vi "Format Vacuum Test Result Table.vi"(10 "Test Configuration":T1, 11 "Test Results":T8) -> (2 "Failure Indexes":i32[](array[numeric]), 3 "Vacuum Results":string[][](array[string]))   [LabVIEW 2014]
uses:
  Tests/Controls/Test Results.ctl
  Tests/Controls/Step Result.ctl
  Tests/Controls/Test Configuration.ctl
  Tests/Controls/Vacuum Test.ctl
  Tests/Controls/Test Timing.ctl
  Tests/Controls/Vaccum Thresholds.ctl
  Tests/Controls/Helium Test.ctl
  Tests/Controls/Helium Thresholds.ctl
  Tests/Controls/Functional Test.ctl
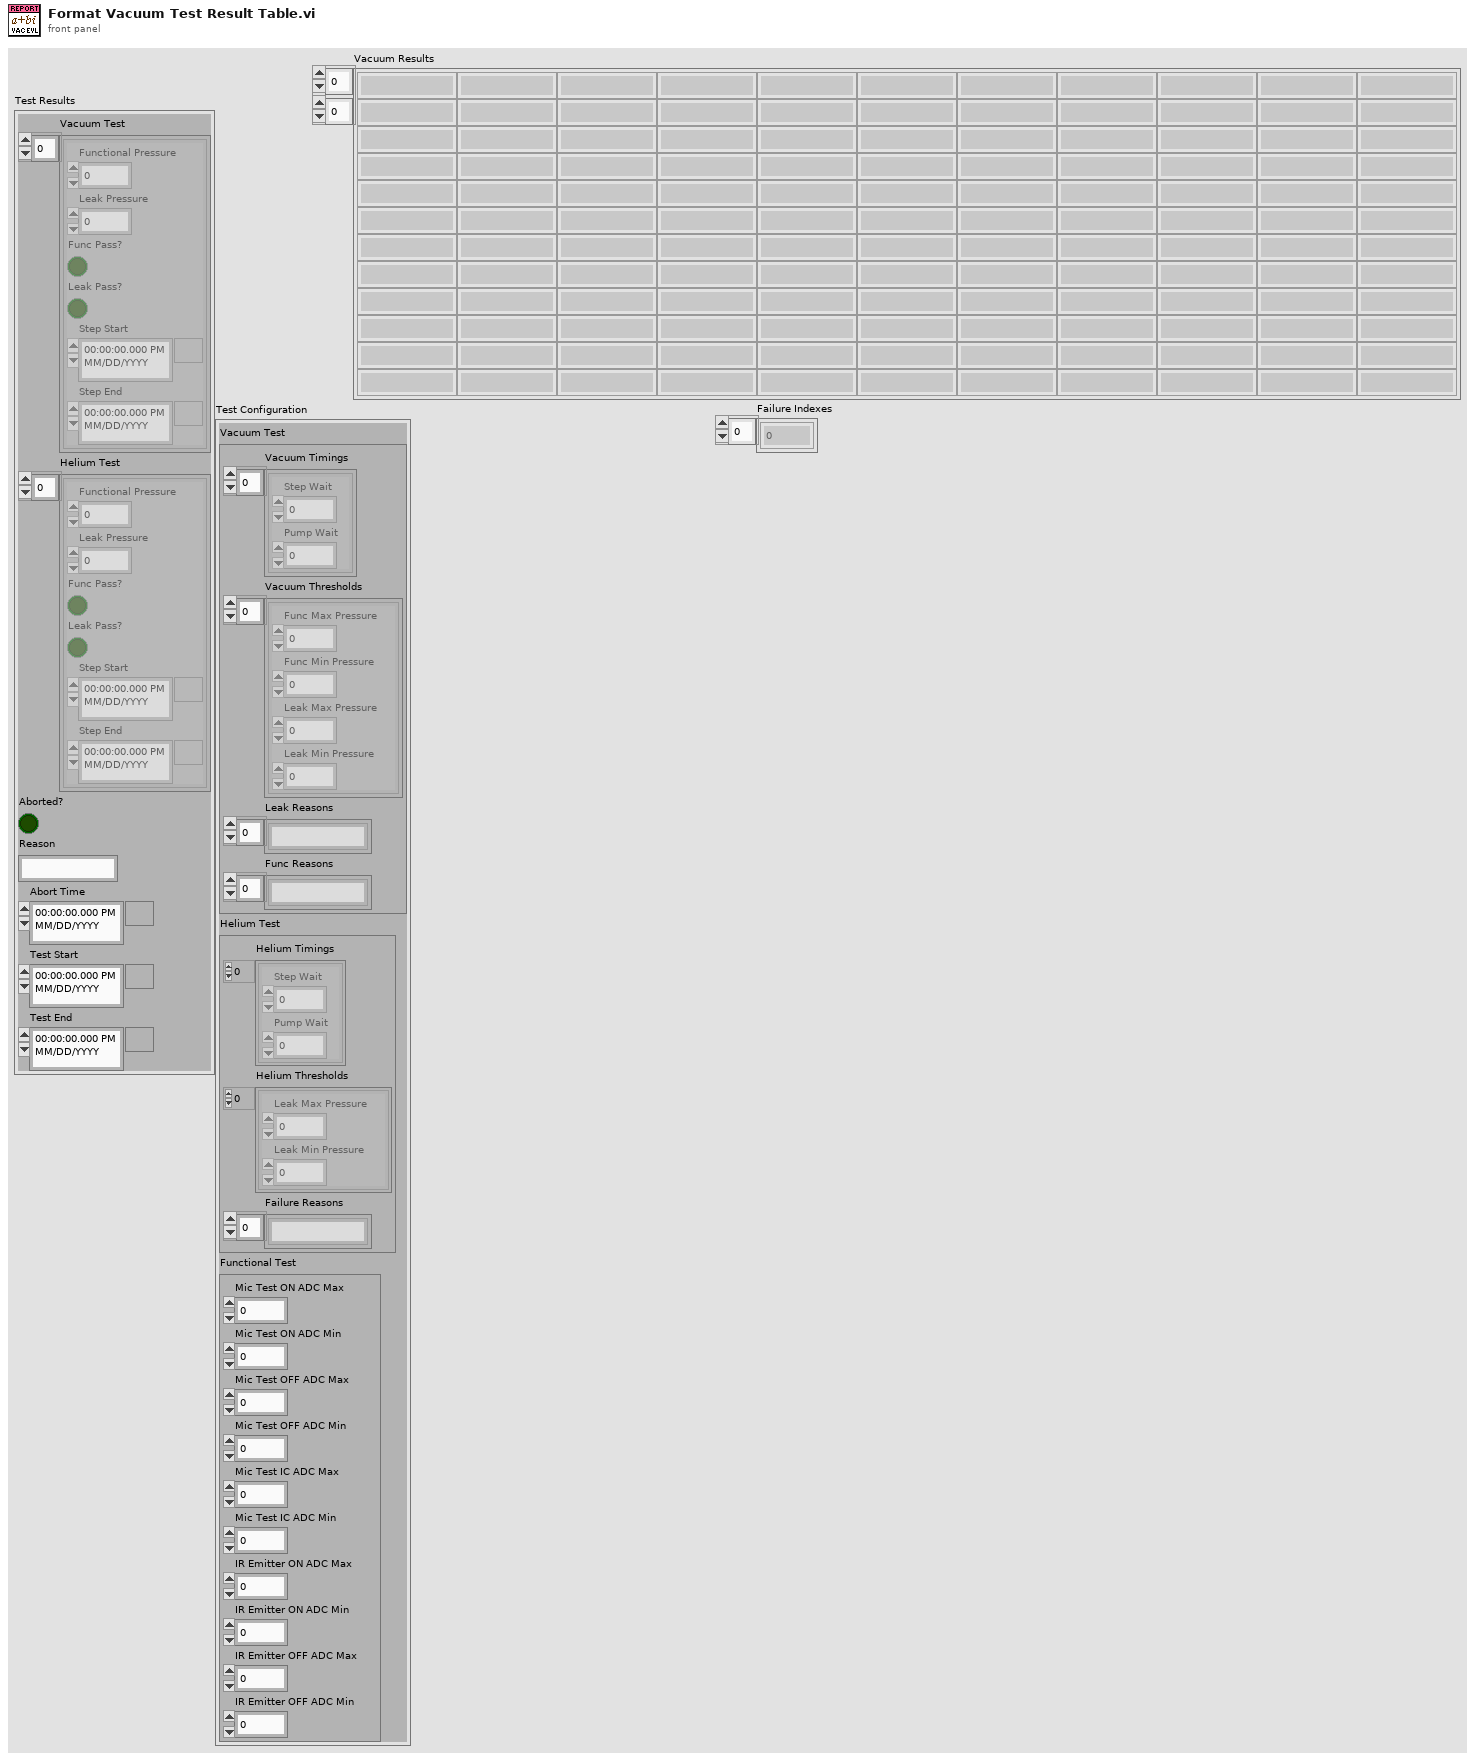
[diagram p1: front panel]
types:
  T1 = typedef "Test Configuration.ctl" = cluster{"Vacuum Test":T2, "Helium Test":T5, "Functional Test":T7}
  T2 = typedef "Vacuum Test.ctl" = cluster{"Vacuum Timings":T3[], "Vacuum Thresholds":T4[], "Leak Reasons":string[], "Func Reasons":string[]}
  T3 = typedef "Test Timing.ctl" = cluster{"Step Wait":dbl, "Pump Wait":dbl}
  T4 = typedef "Vaccum Thresholds.ctl" = cluster{"Func Max Pressure":dbl, "Func Min Pressure":dbl, "Leak Max Pressure":dbl, "Leak Min Pressure":dbl}
  T5 = typedef "Helium Test.ctl" = cluster{"Helium Timings":T3[], "Helium Thresholds":T6[], "Failure Reasons":string[]}
  T6 = typedef "Helium Thresholds.ctl" = cluster{"Leak Max Pressure":dbl, "Leak Min Pressure":dbl}
  T7 = typedef "Functional Test.ctl" = cluster{"Mic Test ON ADC Max":dbl, "Mic Test ON ADC Min":dbl, "Mic Test OFF ADC Max":dbl, "Mic Test OFF ADC Min":dbl, "Mic Test IC ADC Max":dbl, "Mic Test IC ADC Min":dbl, "IR Emitter ON ADC Max":dbl, "IR Emitter ON ADC Min":dbl, "IR Emitter OFF ADC Max":dbl, "IR Emitter OFF ADC Min":dbl}
  T8 = typedef "Test Results.ctl" = cluster{"Vacuum Test":T9[], "Helium Test":T9[], "Aborted?":bool, "Reason":string, "Abort Time":timestamp, "Test Start":timestamp, "Test End":timestamp}
  T9 = typedef "Step Result.ctl" = cluster{"Functional Pressure":dbl, "Leak Pressure":dbl, "Func Pass?":bool, "Leak Pass?":bool, "Step Start":timestamp, "Step End":timestamp}
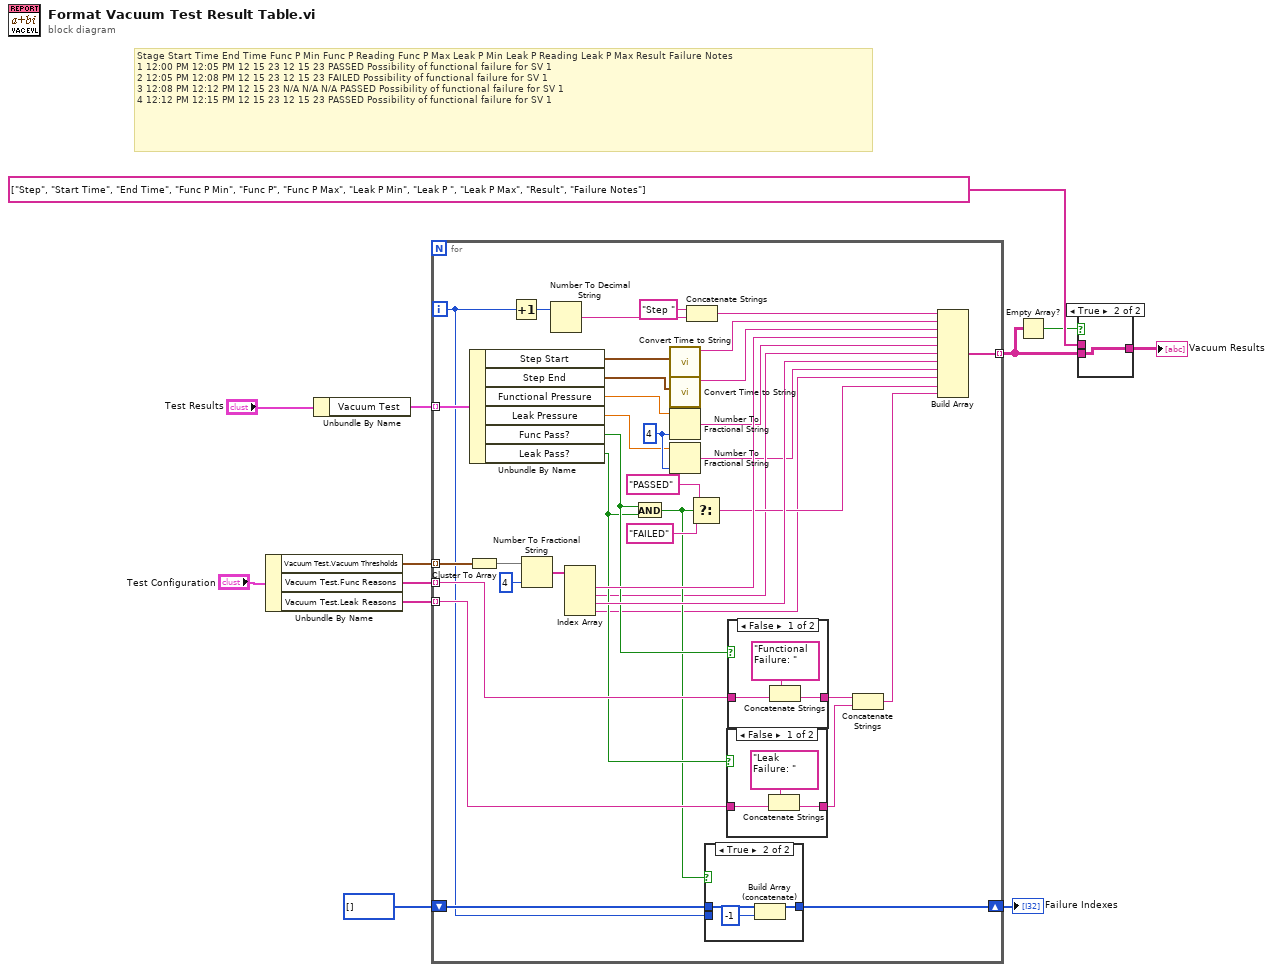
[diagram p0: block diagram]
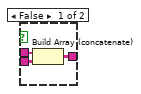
[diagram p2: hidden frame]
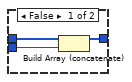
[diagram p3: hidden frame]
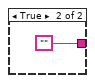
[diagram p4: hidden frame]
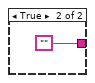
[diagram p5: hidden frame]
diagram:
  # "Stage\tStart Time\tEnd Time\tFunc P Min\tFunc P Reading\tFunc P Max\tLeak P Min\tLeak P Reading\tLeak P Max\tResult\tFailure Notes\n1\t12:00 PM\t12:05 PM\t12\t15\t23\t12\t15\t23\tPASSED\tPossibility of functional failure for SV 1\n2\t12:05 PM\t12:08 PM\t12\t15\t23\t12\t15\t23\tFAILED\tPossibility of functional failure for SV 1\n3\t12:08 PM\t12:12 PM\t12\t15\t23\tN/A\tN/A\tN/A\tPASSED\tPossibility of functional failure for SV 1\n4\t12:12 PM\t12:15 PM\t12\t15\t23\t12\t15\t23\tPASSED\tPossibility of functional failure for SV 1"
  n1 = Unbundle By Name("Test Configuration") -> ("Vacuum Test.Vacuum Thresholds"=w10:T4[], "Vacuum Test.Func Reasons"=w9:string[], "Vacuum Test.Leak Reasons"=w8:string[])
  n2 = Unbundle By Name("Test Results") -> ("Vacuum Test"=w11:T9[])
  n3 = for {
    tunnel: w11 -> [w49] mode=indexing
    tunnel: w10 -> [w45] mode=indexing
    tunnel: w9 -> [w27] mode=indexing
    tunnel: w8 -> [w22] mode=indexing
    tunnel: [w24] -> w3 mode=indexing
    shift-right: [w17] -> w4
    shift-left: i32[] [] -> [w19]
    i -> [w18]
    w33 = i16 4 ("precision (6)")
    n4 = Cluster To Array(cluster=w45) -> (array=w44:dbl[])
    n5 = Unbundle By Name(w49) -> ("Step Start"=w47:timestamp, "Step End"=w46:timestamp, "Functional Pressure"=w41:dbl, "Leak Pressure"=w32:dbl, "Func Pass?"=w28:bool, "Leak Pass?"=w23:bool)
    n6 = Increment(x=w18) -> (x+1=w48:i32)
    n7 = Number To Fractional String(number=w44, precision (6)=i16 4) -> (F-format string=w42:string[])  [unwired: 2 in]
    n8 = Number To Decimal String(number=w48) -> (decimal integer string=w40:string)  [unwired: 1 in]
    n9 = Index Array(array=w42) -> (element #1=w35:string, element #2=w15:string, element #3=w34:string, element #4=w13:string)  [unwired: 4 in]
    n10 = And(x=w28, y=w23) -> (x .and. y?=w20:bool)
    n11 = call "Convert Time to String.vi"("time stamp"=w47) -> ("date/time string"=w37:string)  [unwired: 10 in]
    n12 = call "Convert Time to String.vi"("time stamp"=w46) -> ("date/time string"=w36:string)  [unwired: 10 in]
    n13 = Number To Fractional String(number=w41, precision (6)=w33) -> (F-format string=w16:string)  [unwired: 2 in]
    n14 = Number To Fractional String(number=w32, precision (6)=w33) -> (F-format string=w14:string)  [unwired: 2 in]
    n15 = Concatenate Strings("Step " ("string"), w40) -> (w39:string)
    n16 = Select(t="PASSED", s=w20, f="FAILED") -> (s? t:f=w29:string)
    n17 = case shown="True" w20 {
      tunnel: w19 -> [w52 w55]
      tunnel: w18 -> [w51 _]
      tunnel: [w50 w54] -> w17
      frame False {
        n18 = Build Array (concatenate)(w52, w51) -> (w50:i32[])
      }
      frame True {
        n19 = Build Array (concatenate)(w55, -1) -> (w54:i32[])
      }
    }
    n20 = case shown="False" w23 {
      tunnel: [w57 ""] -> w21
      tunnel: w22 -> [w58 _]
      frame False {
        n21 = Concatenate Strings("Leak Failure: " ("string"), w58) -> (w57:string)
      }
      frame True {
      }
    }
    n22 = case shown="False" w28 {
      tunnel: [w61 ""] -> w26
      tunnel: w27 -> [w62 _]
      frame False {
        n23 = Concatenate Strings("Functional Failure: " ("string"), w62) -> (w61:string)
      }
      frame True {
      }
    }
    n24 = Concatenate Strings(w26, w21) -> (w25:string)
    n25 = Build Array(w39, w37, w36, w35, w16, w15, w34, w14, w13, w29, w25) -> (w24:string[])
  }
  "Failure Indexes" <- w4
  n26 = Empty Array?(array=w3) -> (empty?=w2:bool)
  n27 = case shown="True" w2 {
    tunnel: string[] ["Step", "Start Time", "End Time", "Func P Min", "Func P", "Func P Max", "Leak P Min", "Leak P ", "Leak P Max", "Result", "Failure Notes"] -> [w66 _]
    tunnel: [w65 w67] -> w6
    tunnel: w3 -> [w64 w67]
    frame False {
      n28 = Build Array (concatenate)(w66, w64) -> (w65:string[][])
    }
    frame True {
    }
  }
  "Vacuum Results" <- w6
